vi "234.vi"(10 "FPGAReference":refnum<k20>, 11 "HealthAndStatusDataFIFO in":refnum<class "HealthAndStatusDataFIFO.lvclass">) -> (3 "HealthAndStatusDataFIFO out":refnum<class "HealthAndStatusDataFIFO.lvclass">)   [LabVIEW 2016]
uses:
  HealthAndStatusDataFIFO.lvclass
  D:/Code/ts_M1M3Support/Common_RT_FPGA/IReadU32FIFO/IReadU32FIFO.lvclass
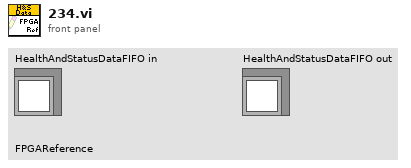
[diagram p1: front panel]
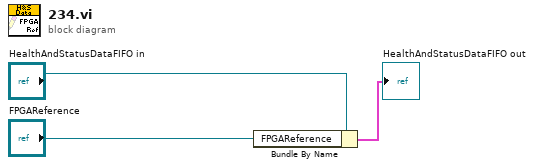
[diagram p0: block diagram]
diagram:
  n1 = Bundle By Name(cluster="HealthAndStatusDataFIFO in", "FPGAReference"="FPGAReference") -> (→"HealthAndStatusDataFIFO out":cluster{})
